vi "hidSPD Close Session.vi"(8 "error in (no error)":errorcluster, 11 "spdDevHandle":T1) -> (0 "error out":errorcluster)   [LabVIEW 2018, in "hidSPDLibForLabView.lvlib"]
uses:
  hidSPDLibForLabView.lvlib
  hidSPD Controls/hidSPD Device Session.ctl
  <vilib>/Utility/error.llb/Error Cluster From Error Code.vi
  <vilib>/ErrorRing/Error Ring.xnode
  hidSPD DLL files/libSPD.dll
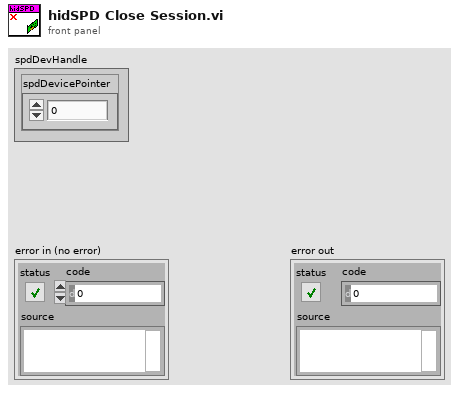
[diagram p1: front panel]
types:
  T1 = typedef "hidSPDLibForLabView.lvlib/hidSPD Device Session.ctl" = cluster{"spdDevicePointer":u64}
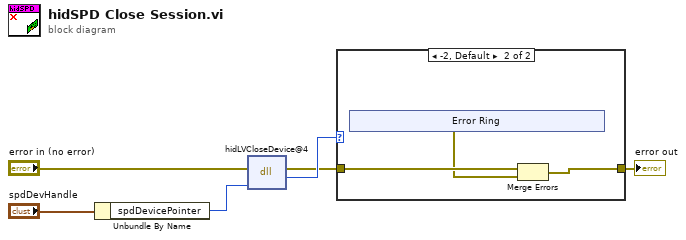
[diagram p0: block diagram]
diagram:
  n1 = Unbundle By Name("spdDevHandle") -> ("spdDevicePointer"=w1:u64)
  n2 = dll-call lib="D:/NextCloud/SPD/hidSPDLibForLabView/hidSPD DLL files/libSPD.dll" fn="hidLVCloseDevice@4"(error in="error in (no error)", "spdDevHandle"=w1) -> (error out=w4:errorcluster, "errorCode"=w5:i32)  [unwired: 3 in, 1 out]
  n3 = case shown="-2, Default" w5 {
    tunnel: w4 -> [w7 w10]
    tunnel: [w7 w8] -> w3
    frame 0 {
    }
    frame -2, Default {
      n4 = xnode "Error Ring"() -> ("error out"=w9:errorcluster)
      n5 = Merge Errors(w10, w9) -> (w8:errorcluster)
    }
  }
  "error out" <- w3
